vi "Radau5_Tolerence Check.vi"(8 "error in (no error)":errorcluster, 10 "Absolute Tolerance":dbl[](array[numeric]), 11 "Relative Tolerance":dbl[](array[numeric])) -> (0 "error out":errorcluster)   [LabVIEW 2017, in "NI_DAE.lvlib"]
uses:
  <vilib>/gmath/NI_DAE.lvlib
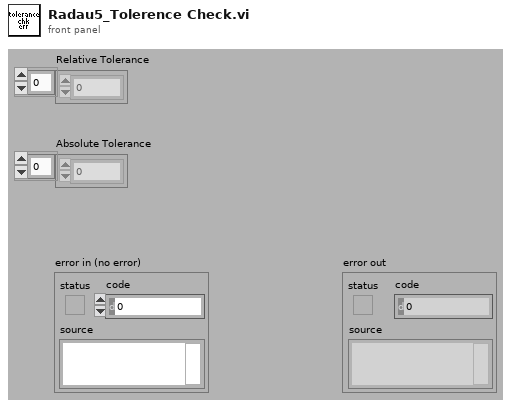
[diagram p1: front panel]
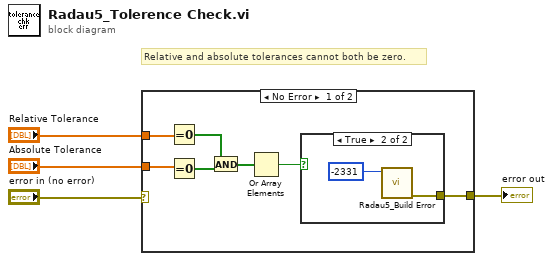
[diagram p0: block diagram]
diagram:
  # "Relative and absolute tolerances cannot both be zero."
  n1 = case shown="No Error" "error in (no error)" {
    selector: "error in (no error)" -> [_ w14]
    tunnel: [w9 w14] -> w4
    tunnel: "Absolute Tolerance" -> [w11 _]
    tunnel: "Relative Tolerance" -> [w10 _]
    frame No Error {
      n2 = Equal To 0?(x=w10) -> (x = 0?=w8:bool[])
      n3 = Equal To 0?(x=w11) -> (x = 0?=w7:bool[])
      n4 = And(x=w8, y=w7) -> (x .and. y?=w6:bool[])
      n5 = Or Array Elements(Boolean array=w6) -> (logical OR=w5:bool)
      n6 = case shown="True" w5 {
        tunnel: [_ w13] -> w9
        frame False {
        }
        frame True {
          n7 = call <vilib>:"Radau5_Build Error.vi"("error code"=-2331 ("error.code")) -> ("error out"=w13:errorcluster)  [unwired: 10 in]
        }
      }
    }
    frame Error {
    }
  }
  "error out" <- w4
